vi "Close.vi"(8 "error in (no error)":errorcluster, 11 "Serial in":refnum<class "Serial.lvclass">) -> (0 "error out":errorcluster, 3 "Serial out":refnum<class "Serial.lvclass">)   [LabVIEW 2021, in "Serial.lvclass"]
uses:
  Serial.lvclass
  Serial.lvclass/Serial.ctl
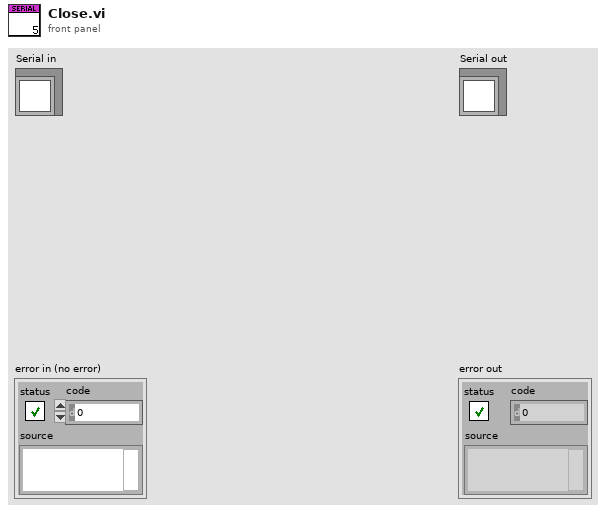
[diagram p1: front panel]
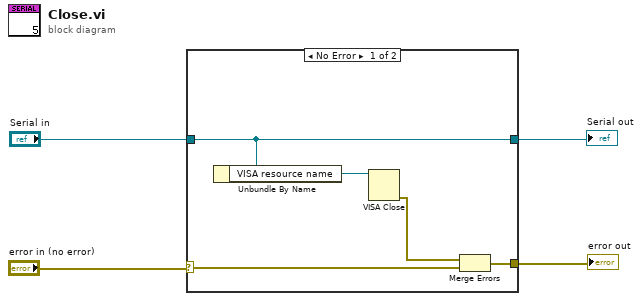
[diagram p0: block diagram]
diagram:
  n1 = case shown="No Error" "error in (no error)" {
    selector: "error in (no error)" -> [w9 w10]
    tunnel: "Serial in" -> [w5 w11]
    tunnel: [w6 w10] -> w2
    tunnel: [w5 w11] -> w1
    frame No Error {
      n2 = Unbundle By Name(w5) -> ("VISA resource name"=w8:refnum<visa-resource-name>)
      n3 = VISA Close(VISA resource name=w8) -> (error out=w7:errorcluster)  [unwired: 1 in]
      n4 = Merge Errors(w7, w9) -> (w6:errorcluster)
    }
    frame Error {
    }
  }
  "error out" <- w2
  "Serial out" <- w1
